vi "Stop Logs.vi"(8 "error in (no error)":errorcluster, 11 "Historian Logger in":refnum<class "Historian Logger.lvclass">) -> (0 "error out":errorcluster, 3 "Historian Logger out":refnum<class "Historian Logger.lvclass">)   [LabVIEW 2020, in "VolatusHistorian.lvlib" / "Historian Logger.lvclass"]
uses:
  Historian Logger.lvclass
  Historian Logger.lvclass/Historian Logger.ctl
  VolatusData/VolatusData.lvlib
  VolatusErrorUtilities/MultiErrors/MultiErrors.lvclass
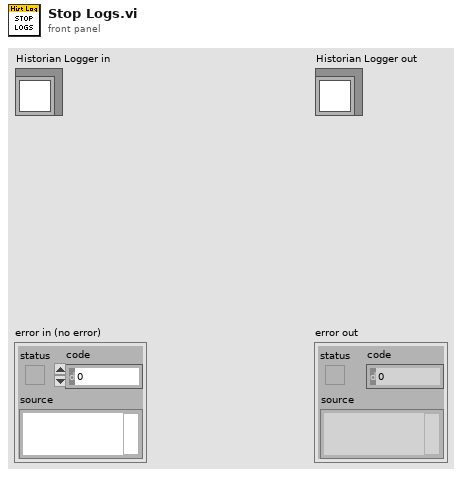
[diagram p1: front panel]
types:
  T1 = typedef "VolatusHistorian.lvlib/Historian Logger.lvclass/Group Info.ctl" = cluster{"Buffer":refnum<class "Group Buffer DBL.lvclass">, "Logger":refnum<class "MessageQ.lvclass">, "Group":refnum<class "Group DBL.lvclass">, "Last Timestamp":dbl, "State":T2}
  T2 = typedef "VolatusData.lvlib/Logger State.ctl" = enum16{"Unknown", "Idle", "Preparing", "Ready", "Logging", "Stopping"}
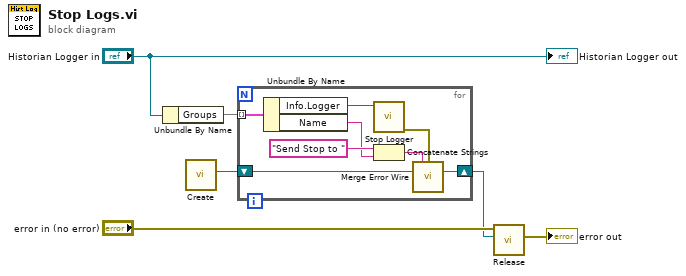
[diagram p0: block diagram]
diagram:
  n1 = Unbundle By Name("Historian Logger in") -> ("Groups"=w4:map{string, T1})
  n2 = call "Create.vi"() -> ("MultiErrors out"=w3:refnum<class "MultiErrors.lvclass">)  [unwired: 11 in]
  n3 = for {
    tunnel: w4 -> [w14] mode=indexing
    shift-right: [w11] -> w1
    shift-left: w3 -> [w12]
    n4 = Unbundle By Name(w14) -> ("Info.Logger"=w13:refnum<class "MessageQ.lvclass">, "Name"=w8:string)
    n5 = call "Stop Logger.vi"("MsgQ in"=w13) -> ("error out"=w10:errorcluster)  [unwired: 9 in, 1 out]
    n6 = Concatenate Strings("Send Stop to ", w8) -> (w7:string)
    n7 = call "Merge Error Wire.vi"("Local Context (None)"=w7, "error in (no error)"=w10, "MultiErrors in"=w12) -> ("MultiErrors out"=w11:refnum<class "MultiErrors.lvclass">)  [unwired: 12 in]
  }
  n8 = call "Release.vi"("MultiErrors in"=w1, "Upstream Error (None)"="error in (no error)") -> ("error out"=→"error out":errorcluster)  [unwired: 9 in]
  "Historian Logger out" <- "Historian Logger in"
